vi "ziExample1-PollData.vi"(0 "Address":string="DEV", 1 "stop":bool, 5 "Save":bool) -> (17 "theta (deg)":dbl[](array[numeric]), 20 "Selected Device":string, 21 "Demod R (V)":dbl format="%_4p", 22 "Demod Phi (rad)":dbl format="%.3p", 23 "Spectral Density\nVrms/sqrt(Hz)":dbl=1.331104953906021e-08 format="%0.2p", 24 "Savedas":string, 25 "Demod Sample Out":T3 {"Aux In 1 (V)" format="%#_5p"; "Aux In 0 (V)" format="%#_5p"; "X (Vrms)" format="%#_5p"; "Y (Vrms)" format="%#_5p"; "Osc Phase (rad)" format="%#.3g"}, 26 "DIO Out":T2, 27 "AuxIn Out":T1)   [LabVIEW 2016]
doc: "Control a Zurich instrument device via the LabOne Labview API. \nRequirements: Zurich Instruments MFLI, HF2 or UHFLI \nThis example polls data from the instrument.\n\n© Zurich Instruments AG, www.zhinst.com"
uses:
  <instrlib>/Zurich Instruments LabOne/Public/Data/ziTypeDemodSampleEx.ctl
  <instrlib>/Zurich Instruments LabOne/Public/Data/ziTypeAuxInSample.ctl
  <instrlib>/Zurich Instruments LabOne/Public/Configure/ziSetValueDoubleArray.vi
  <instrlib>/Zurich Instruments LabOne/Public/Configure/ziGetValueDouble.vi
  <instrlib>/Zurich Instruments LabOne/Public/Data/ziGetEventAuxInSample.vi
  <instrlib>/Zurich Instruments LabOne/Public/Data/ziGetEventDemodSample.vi
  <instrlib>/Zurich Instruments LabOne/Public/Data/ziGetEventDIOSample.vi
  <instrlib>/Zurich Instruments LabOne/Zurich Instruments LabOne.lvlib
panel:
  out "Error Out":errorcluster
  in  "Saveas":string
  in  "Edge":u16(ring)=1 items=["Off", "Rising Edge", "Falling Edge", "Both Edges"]
  in  "DIO Channel":u16(ring) items=["Continous"=0, "DIO 0 / Tigger 3"=1, "DIO 1 / Tigger 4"=4, "DIO 0|1 / Tigger 3|4"=5]
  in  "binSave":bool caption="Binary Save"
  out "Buffer Overflow":bool
  out "Demod sample":dbl[](graph)
  out "DIO":u32[](graph)
  out "AUX Input":dbl[](graph)
  # "ziExample-PollData.vi\nRequirements: HF2, UHFLI or MFLI\nsee block diagram for VI description"
  # "Tested Instruments:\n- MFLI\n- HF2LI\n- UHFLI"
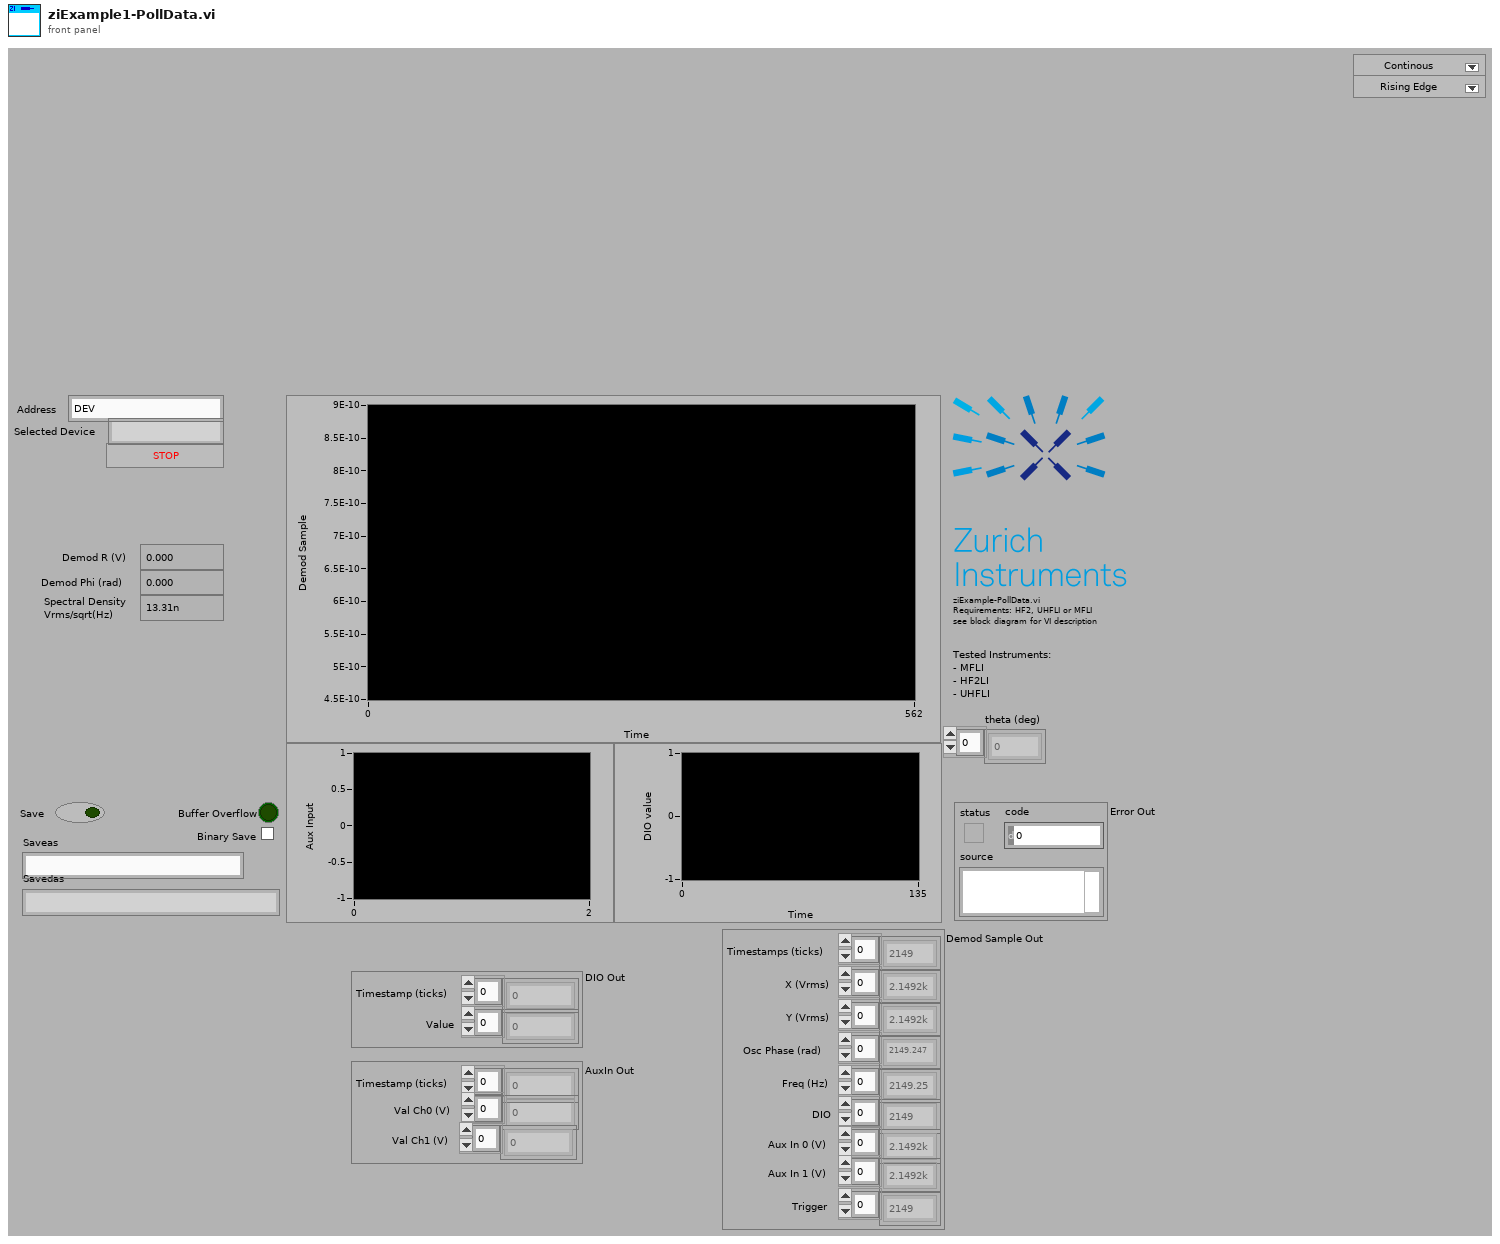
[diagram p1: front panel]
types:
  T1 = typedef "Zurich Instruments LabOne.lvlib/ziTypeAuxInSample.ctl" = cluster{"Timestamp (ticks)":u64[], "Val Ch0 (V)":dbl[], "Val Ch1 (V)":dbl[]}
  T2 = cluster{"Timestamp (ticks)":u64[], "Value":u32[]}
  T3 = typedef "Zurich Instruments LabOne.lvlib/ziTypeDemodSampleEx.ctl" = cluster{"Timestamps (ticks)":u64[], "X (Vrms)":dbl[], "Y (Vrms)":dbl[], "Osc Phase (rad)":dbl[], "Freq (Hz)":dbl[], "DIO":u32[], "Aux In 0 (V)":dbl[], "Aux In 1 (V)":dbl[], "Trigger":u32[]}
  T4 = typedef "Zurich Instruments LabOne.lvlib/ziTypeHandle.ctl" = cluster{"handleValid":bool, "Conn":u64, "Path Prefix":string, "Handle":u64, "Connected":bool, "Clockbase(s)":dbl}
  T5 = enum16{"open", "replace", "create", "open or create", "replace or create", "replace or create with confirmation"}
  T6 = typedef "Zurich Instruments LabOne.lvlib/ziTypePollType.ctl" = enum16{"NONE", "DOUBLE_DATA", "INTEGER_DATA", "DEMOD_SAMPLE", "SCOPE_WAVE_HF2", "AUXIN_SAMPLE", "DIO_SAMPLE", "BYTE_ARRAY", "PWA_WAVE", "9", "10", "11", "12", "13", "14", "15", "TREE_CHANGE_DEPRI", "17", "ERROR", "19", "20", "21", "22", "23", "24", "25", "26", "27", "28", "29", "30", "31", "DOUBLE_DATA_TS", "INTEGER_DATA_TS", "34", "SCOPE_WAVE", "SCOPE_WAVE_EX", "37", "BYTE_ARRAY_TS", "39", "40", "41", "42", "43", "44", "45", "CNT_DATA", "47", "TREE_CHANGE", "49", "50", "51", "52", "53", "54", "55", "56", "57", "58", "59", "60", "61", "62", "63", "SWEEPER_DATA", "SPECTRUM_DATA", "ADVISOR_DATA", "VECTOR_DATA", "IMP_DATA"}
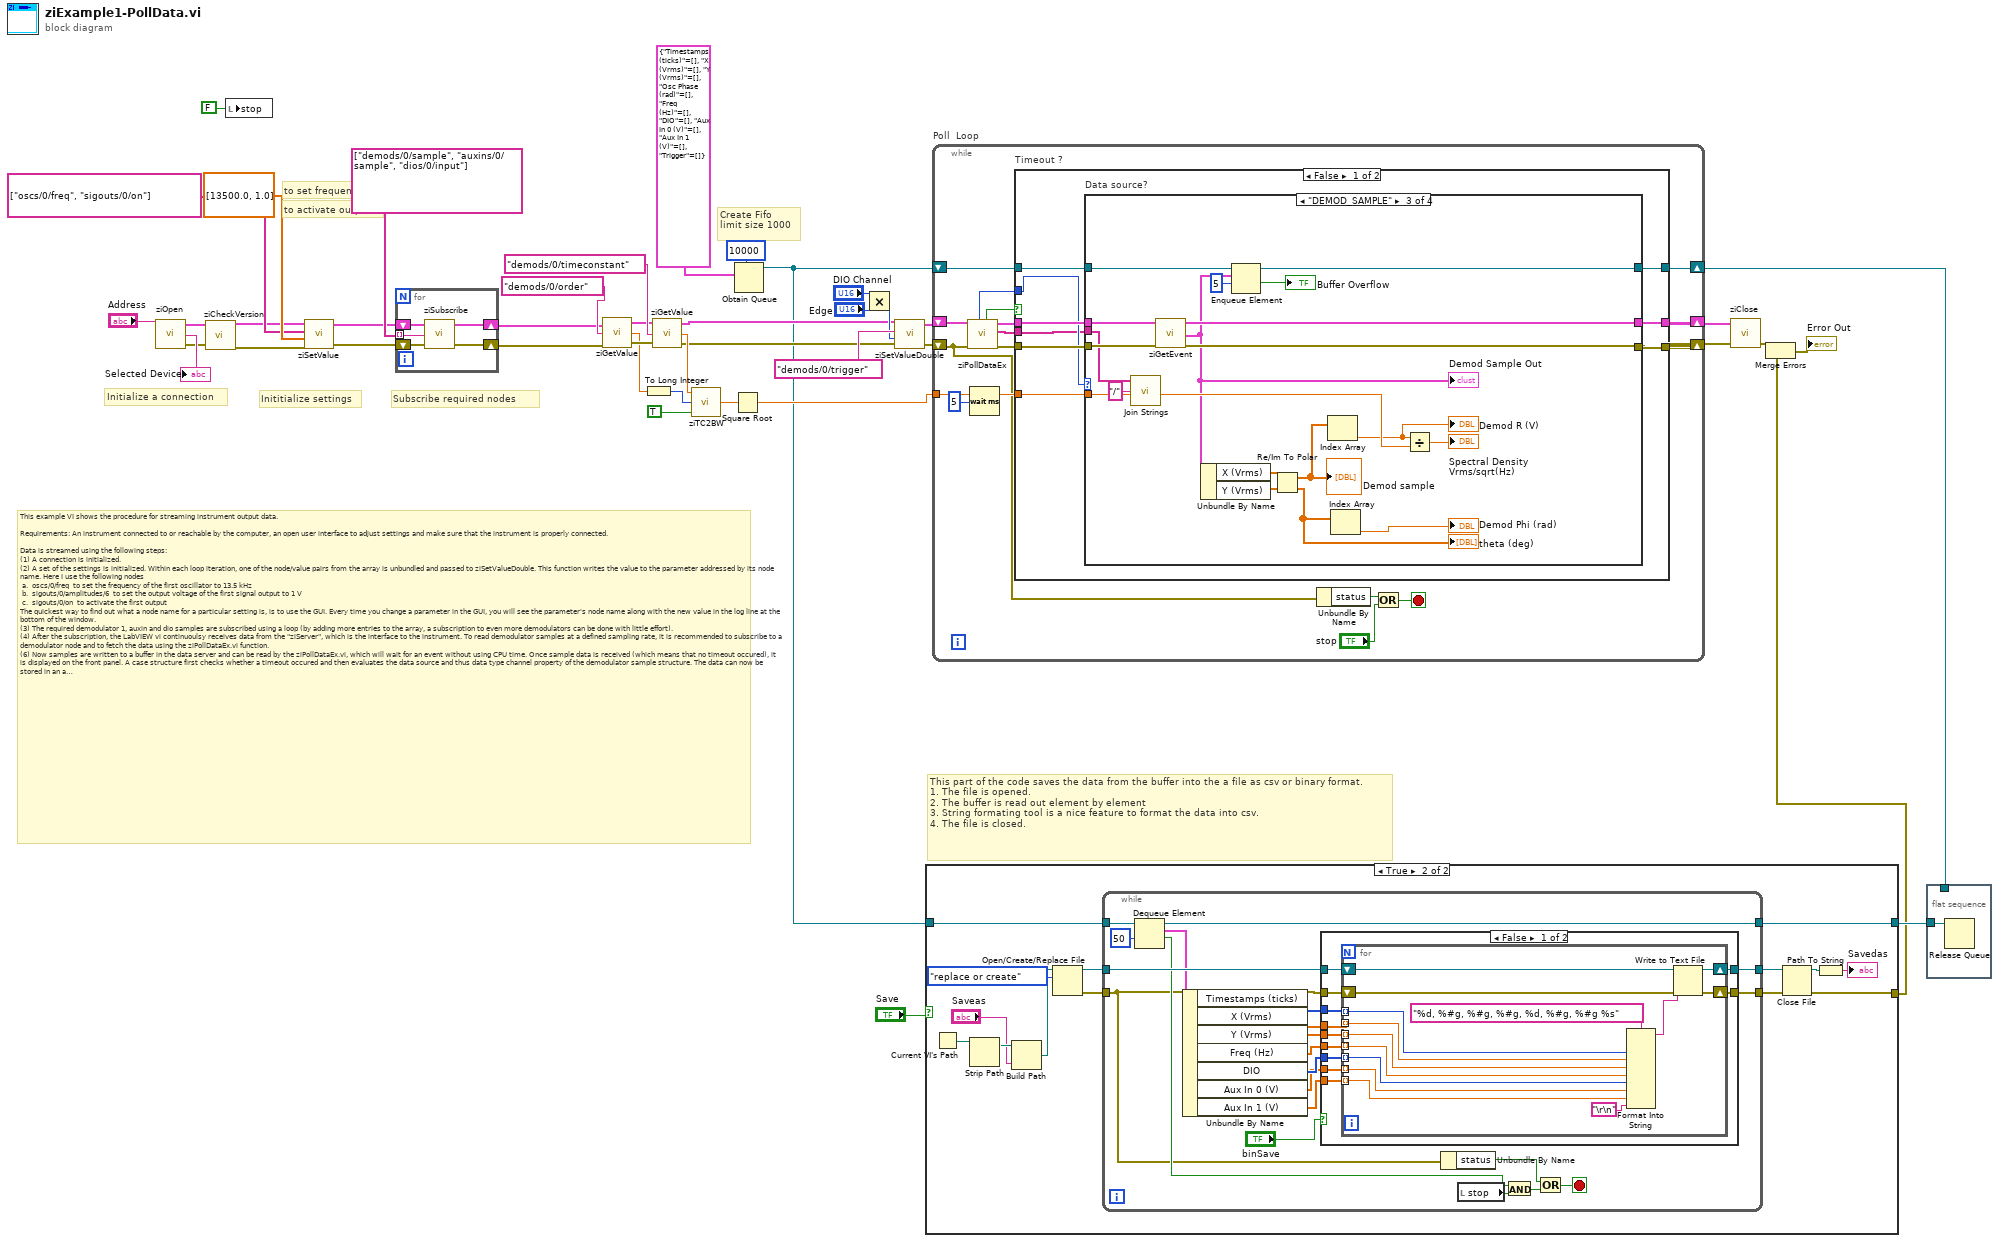
[diagram p0: block diagram]
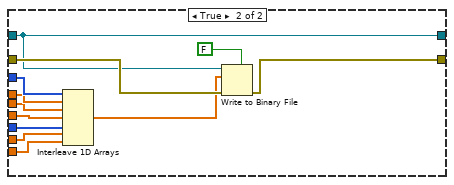
[diagram p3: hidden frame]
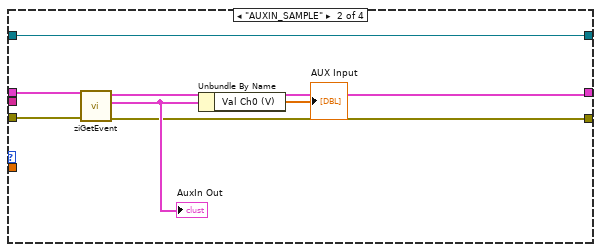
[diagram p5: hidden frame]
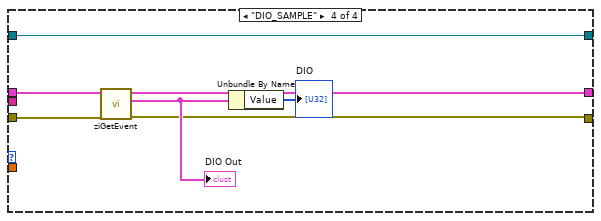
[diagram p6: hidden frame]
diagram:
  # "This part of the code saves the data from the buffer into the a file as csv or binary format. \n1. The file is opened.\n2. The buffer is read out element by element\n3. String formating tool is a nice feature to format the data into csv.\n4. The file is closed."
  # "Create Fifo\nlimit size 1000"
  # "to activate output"
  # "to set frequency"
  # "Inititialize settings"
  # "Initialize a connection"
  # "Subscribe required nodes"
  # "This example VI shows the procedure for streaming instrument output data.\n\nRequirements: An instrument connected to or reachable by the computer, an open user interface to adjust settings and make sure that the instrument is properly connected. \n\nData is streamed using the following steps:\n(1) A connection is initialized.\n(2) A set of the settings is initialized. Within each loop iteration, one of the node/value pairs from the array is unbundled and passed to ziSetValueDouble. This function writes the value to the parameter addressed by its node name. Here I use the following nodes\n a. \toscs/0/freq \tto set the frequency of the first oscillator to 13.5 kHz\n b. \tsigouts/0/amplitudes/6 \tto set the output voltage of the first signal output to 1 V\n c. \tsigouts/0/on \tto activate the first output\nThe quickest way to find out what a node name for a particular setting is, is to use the GUI. Every time you change a parameter in the GUI, you will see the parameter's node name along with the new value in the log line at the bottom of the window. \n(3) The required demodulator 1, auxin and dio samples are subscribed using a loop (by adding more entries to the array, a subscription to even more demodulators can be done with little effort).\n(4) After the subscription, the LabVIEW vi continuoulsy receives data from the \"ziServer\", which is the interface to the instrument. To read demodulator samples at a defined sampling rate, it is recommended to subscribe to a demodulator node and to fetch the data using the ziPollDataEx.vi function. \n(6) Now samples are written to a buffer in the data server and can be read by the ziPollDataEx.vi, which will wait for an event without using CPU time. Once sample data is received (which means that no timeout occured), it is displayed on the front panel. A case structure first checks whether a timeout occured and then evaluates the data source and thus data type channel property of the demodulator sample structure. The data can now be stored in an array or a queue or be shown in a waveform chart. \n(7) Finally, the connection is closed. \n \n© Zurich Instruments AG, 2016, www.zhinst.com"
  n1 = call <instrlib>:"ziOpen.vi"("Address"="Address") -> ("Error Out"=w3:errorcluster, "Selected Device"=→"Selected Device":string, "HandleOut"=w4:T4)  [unwired: 1 in, 2 out]
  n2 = call <instrlib>:"ziCheckVersion.vi"("Handle In"=w4, "Error In"=w3) -> ("Handle Out"=w1:T4, "Error Out"=w2:errorcluster)  [unwired: 11 in, 1 out]
  n3 = local write "stop"(FALSE ("stop")) -> ()
  n4 = call-poly <instrlib>:"ziSetValue.vi"("Error In"=w2, "Values"=dbl[] [13500.0, 1.0], "Paths"=string[] ["oscs/0/freq", "sigouts/0/on"], "Handle In"=w1) -> ("Error Out"=w40:errorcluster, "Handle Out"=w41:T4)  [unwired: 1 in]
  n5 = for {
    shift-right: [w48] -> w24
    shift-left: w41 -> [w46]
    shift-right: [w47] -> w23
    shift-left: w40 -> [w45]
    tunnel: string[] ["demods/0/sample", "auxins/0/sample", "dios/0/input"] -> [w44] mode=indexing
    n6 = call <instrlib>:"ziSubscribe.vi"("error in"=w45, "Path ()"=w44, "Handle In"=w46) -> ("error out"=w47:errorcluster, "Handle Out"=w48:T4)  [unwired: 1 in]
  }
  n7 = call-poly <instrlib>:"ziGetValue.vi"("error in"=w23, "Path"="demods/0/order", "Handle in"=w24) -> ("error out"=w30:errorcluster, "Value"=w29:dbl, "Handle out"=w31:T4)
  n8 = To Long Integer(number=w29) -> (32bit integer=w28:i32)
  n9 = call-poly <instrlib>:"ziGetValue.vi"("error in"=w30, "Path"="demods/0/timeconstant", "Handle in"=w31) -> ("error out"=w11:errorcluster, "Value"=w27:dbl, "Handle out"=w12:T4)
  n10 = call <instrlib>:"ziTC2BW.vi"("Eq BW (F)"=TRUE ("Eq BW"), "Order (1)"=w28, "TC (s)"=w27) -> ("BW (Hz)"=w26:dbl)
  n11 = Square Root(x=w26) -> (sqrt(x)=w22:dbl)
  n12 = Obtain Queue(max queue size (-1, unlimited)=10000, element data type=T3 {"Timestamps (ticks)"=[], "X (Vrms)"=[], "Y (Vrms)"=[], "Osc Phase (rad)"=[], "Freq (Hz)"=[], "DIO"=[], "Aux In 0 (V)"=[], "Aux In 1 (V)"=[], "Trigger"=[]} ("Demod Sample Out")) -> (queue out=w10:refnum<queue>)  [unwired: 3 in, 2 out]
  n13 = Multiply(x="DIO Channel", y="Edge") -> (x*y=w17:u16)
  n14 = call <instrlib>:"ziSetValueDouble.vi"("Error In"=w11, "Value"=w17, "Path"="demods/0/trigger", "Handle In"=w12) -> ("Error Out"=w14:errorcluster, "Handle Out"=w13:T4)  [unwired: 1 in]
  n15 = case shown="True" "Save" {
    tunnel: w10 -> [w49 w63]
    tunnel: [w49 w58] -> w20
    tunnel: [_ w50] -> w5
    frame False {
    }
    frame True {
      n16 = Current VI's Path() -> (path=w54:path)
      n17 = Strip Path(path=w54) -> (stripped path=w53:path)  [unwired: 1 out]
      n18 = Build Path(base path=w53, name or relative path="Saveas") -> (appended path=w51:path)
      n19 = Open/Create/Replace File(file path (use dialog)=w51, operation (0:open)=T5."replace or create") -> (refnum out=w61:refnum<file>, error out=w62:errorcluster)  [unwired: 4 in, 1 out]
      n20 = while {
        tunnel: w62 -> [w66]
        tunnel: w61 -> [w77]
        tunnel: [w76] -> w60
        tunnel: [w75] -> w59
        tunnel: [w70] -> w58
        tunnel: w63 -> [w72]
        stop <- w64 stop-if-true
        n21 = Dequeue Element(queue=w72, timeout in ms (-1)=50) -> (queue out=w70:refnum<queue>, element=w73:T3, timed out?=w71:bool)  [unwired: 1 in, 1 out]
        n22 = Unbundle By Name(w73) -> ("Timestamps (ticks)"=w84:u64[], "X (Vrms)"=w81:dbl[], "Y (Vrms)"=w83:dbl[], "Freq (Hz)"=w82:dbl[], "DIO"=w80:u32[], "Aux In 0 (V)"=w79:dbl[], "Aux In 1 (V)"=w78:dbl[])
        n23 = case shown="False" "binSave" {
          tunnel: w84 -> [w95 w117]
          tunnel: w83 -> [w94 w115]
          tunnel: w82 -> [w93 w114]
          tunnel: w81 -> [w92 w116]
          tunnel: w80 -> [w91 w113]
          tunnel: w79 -> [w90 w112]
          tunnel: w78 -> [w89 w111]
          tunnel: w66 -> [w88 w120]
          tunnel: w77 -> [w87 w118]
          tunnel: [w86 w119] -> w76
          tunnel: [w85 w118] -> w75
          frame False {
            n24 = for {
              tunnel: w95 -> [w103] mode=indexing
              tunnel: w94 -> [w101] mode=indexing
              tunnel: w92 -> [w102] mode=indexing
              shift-right: [w108] -> w85
              shift-left: w87 -> [w109]
              tunnel: w93 -> [w100] mode=indexing
              shift-right: [w107] -> w86
              shift-left: w88 -> [w106]
              tunnel: w91 -> [w98] mode=indexing
              tunnel: w90 -> [w97] mode=indexing
              tunnel: w89 -> [w99] mode=indexing
              n25 = Format Into String(format string="%d, %#g, %#g, %#g, %d, %#g, %#g %s", w103, w102, w101, w100, w98, w97, w99, "\r\n") -> (resulting string=w96:string)  [unwired: 2 in, 1 out]
              n26 = Write to Text File(file (use dialog)=w109, text=w96, error in=w106) -> (refnum out=w108:refnum<file>, error out=w107:errorcluster)  [unwired: 2 out]
            }
          }
          frame True {
            n27 = Interleave 1D Arrays(w117, w116, w115, w114, w113, w112, w111) -> (w110:dbl[])
            n28 = Write to Binary File(file (use dialog)=w118, data=w110, error in=w120, 5:FALSE ("prepend array or string size? (T)")) -> (error out=w119:errorcluster)  [unwired: 4 out]
          }
        }
        n29 = Unbundle By Name(w66) -> ("status"=w67:bool)
        n30 = local read "stop"() -> (w69:bool)
        n31 = And(x=w71, y=w69) -> (x .and. y?=w65:bool)
        n32 = Or(x=w67, y=w65) -> (x .or. y?=w64:bool)
      }
      n33 = Close File(refnum=w59, error in=w60) -> (path=w55:path, error out=w50:errorcluster)
      n34 = Path To String(path=w55) -> (string=→"Savedas":string)
    }
  }
  n35 = while "Poll  Loop" {
    shift-right: [w137] -> w43
    shift-left: w13 -> [w127]
    shift-right: [w133] -> w21
    shift-left: w14 -> [w124]
    shift-right: [w130] -> w9
    shift-left: w10 -> [w131]
    tunnel: w22 -> [w129]
    stop <- w122 stop-if-true
    n36 = call <instrlib>:"ziPollDataEx.vi"("error in"=w124, "Handle In"=w127) -> ("error out"=w134:errorcluster, "PathArray"=w126:string[], "Handle Out"=w136:T4, "Timed Out"=w135:bool, "ziValueType"=w132:T6)  [unwired: 2 in, 3 out]
    n37 = Wait (ms)(milliseconds to wait=u32 5) -> ()  [unwired: 1 out]
    n38 = case "Timeout ?" shown="False" w135 {
      tunnel: w136 -> [w146 w185]
      tunnel: [w145 w185] -> w137
      tunnel: w134 -> [w144 w184]
      tunnel: [w143 w184] -> w133
      tunnel: w132 -> [w139 _]
      tunnel: [w142 w183] -> w130
      tunnel: w131 -> [w141 w183]
      tunnel: w129 -> [w140 _]
      tunnel: w126 -> [w138 _]
      frame False {
        n39 = case "Data source?" shown="\"DEMOD_SAMPLE\"" w139 {
          tunnel: w146 -> [w149 w156 w175 w182]
          tunnel: [w149 w154 w174 w181] -> w145
          tunnel: w144 -> [w148 w153 w173 w179]
          tunnel: [w148 w152 w172 w178] -> w143
          tunnel: [w147 w151 w171 w177] -> w142
          tunnel: w141 -> [w147 w151 w170 w177]
          tunnel: w140 -> [_ _ w169 _]
          tunnel: w138 -> [_ _ w158 _]
          frame Default {
          }
          frame "AUXIN_SAMPLE" {
            n40 = call-poly <instrlib>:"ziGetEvent.vi"("Error In"=w153, "Handle In"=w156) -> ("Error Out"=w152:errorcluster, "AuxIn Out"=w155:T1, "Handle Out"=w154:T4)  [unwired: 7 in]
            "AuxIn Out" <- w155
            n41 = Unbundle By Name(w155) -> ("Val Ch0 (V)"=→"AUX Input":dbl[])
          }
          frame "DEMOD_SAMPLE" {
            n42 = call <vilib>:"Join Strings.vi"("Separator (,)"="/", "Strings In"=w158) -> ()  [unwired: 1 in, 1 out]
            n43 = call-poly <instrlib>:"ziGetEvent.vi"("Error In"=w173, "Handle In"=w175) -> ("Error Out"=w172:errorcluster, "Demod Sample Out"=w166:T3, "Handle Out"=w174:T4)  [unwired: 7 in]
            "Demod Sample Out" <- w166
            n44 = Unbundle By Name(w166) -> ("X (Vrms)"=w168:dbl[], "Y (Vrms)"=w167:dbl[])
            n45 = Enqueue Element(queue=w170, element=w166, timeout in ms (-1)=5) -> (queue out=w171:refnum<queue>, timed out?=→"Buffer Overflow":bool)  [unwired: 1 in, 1 out]
            n46 = Re/Im To Polar(2:w167, 3:w168) -> (0:w161:dbl[], 1:w162:dbl[])
            "Demod sample" <- w162
            "theta (deg)" <- w161
            n47 = Index Array(array=w162) -> (element=w159:dbl)  [unwired: 1 in]
            "Demod R (V)" <- w159
            n48 = Index Array(array=w161) -> (element=→"Demod Phi (rad)":dbl)  [unwired: 1 in]
            n49 = Divide(x=w159, y=w169) -> (x/y=→"Spectral Density\nVrms/sqrt(Hz)":dbl)
          }
          frame "DIO_SAMPLE" {
            n50 = call-poly <instrlib>:"ziGetEvent.vi"("Error In"=w179, "Handle In"=w182) -> ("Error Out"=w178:errorcluster, "DIO Out"=w180:T2, "Handle Out"=w181:T4)  [unwired: 7 in]
            "DIO Out" <- w180
            n51 = Unbundle By Name(w180) -> ("Value"=→"DIO":u32[])
          }
        }
      }
      frame True {
        # "Timeout, no action."
      }
    }
    n52 = Unbundle By Name(w124) -> ("status"=w125:bool)
    n53 = Or(x=w125, y="stop") -> (x .or. y?=w122:bool)
  }
  n54 = call <instrlib>:"ziClose.vi"("Error In"=w21, "Handle In"=w43) -> ("Error Out"=w7:errorcluster)  [unwired: 3 out]
  n55 = Merge Errors(w7, w5) -> (→"Error Out":errorcluster)
  n56 = flat-sequence {
    tunnel: w20 -> [w186]
    tunnel: w9 -> [_]
    frame #0 {
      n57 = Release Queue(queue=w186) -> ()  [unwired: 2 in, 3 out]
    }
  }
